vi "Filter Repeat Barrels.vi"(8 "error in (no error)":errorcluster, 10 "Barrel Array":T1(array[cluster])) -> (0 "error out":errorcluster, 2 "Observed LM Array":T1(array[cluster]))   [LabVIEW 2009]
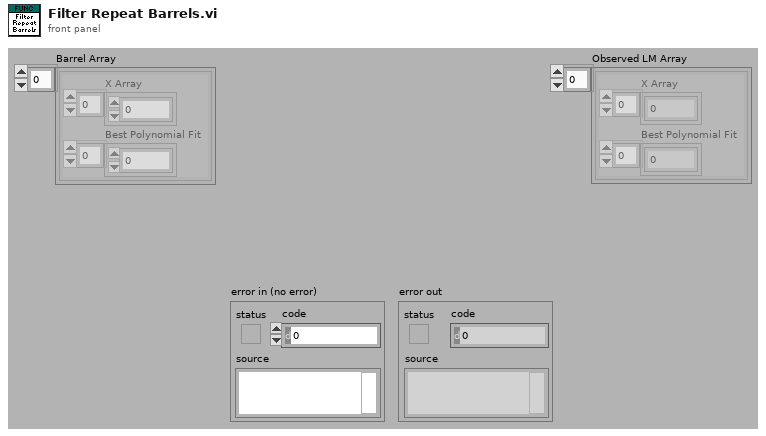
[diagram p1: front panel]
types:
  T1 = cluster{"X Array":dbl[], "Best Polynomial Fit":dbl[]}[]
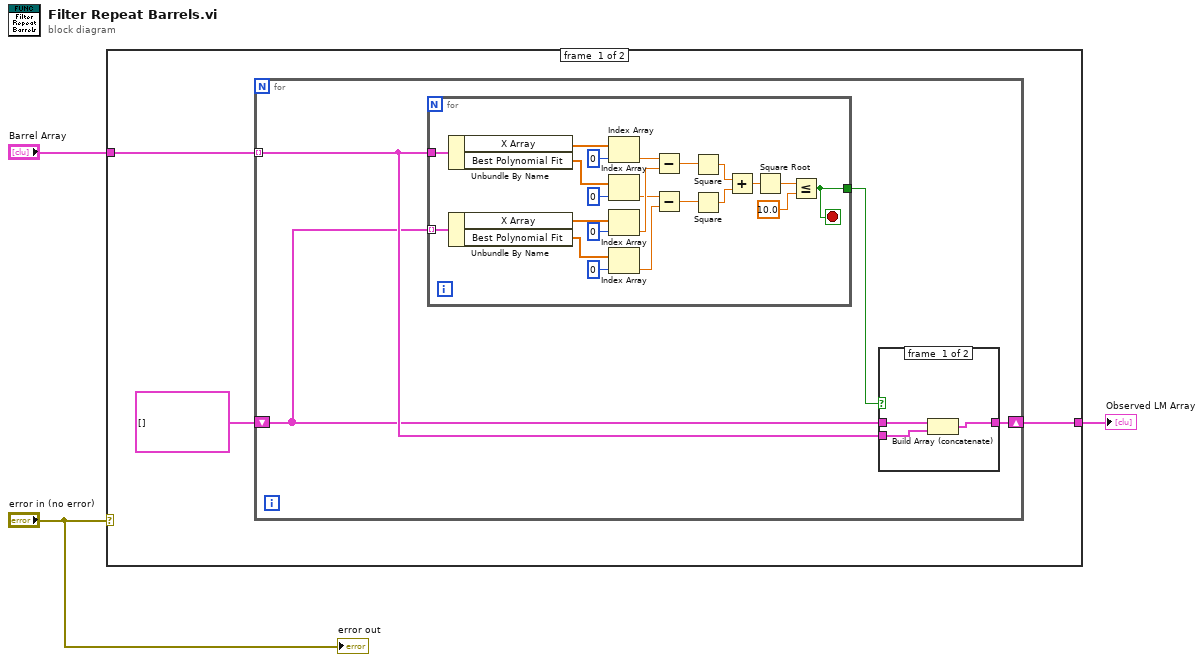
[diagram p0: block diagram]
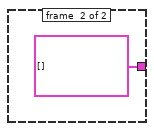
[diagram p3: hidden frame]
diagram:
  n1 = case shown="No Error" "error in (no error)" {
    tunnel: "Barrel Array" -> [w5 _]
    tunnel: [w4 T1 []] -> w2
    frame #0 {
      n2 = for {
        tunnel: w5 -> [w10] mode=indexing
        shift-right: [w7] -> w4
        shift-left: T1 [] -> [w8]
        n3 = for {
          tunnel: w8 -> [w35] mode=indexing
          tunnel: w10 -> [w36]
          tunnel: [w15] -> w9
          stop <- w15 stop-if-true
          n4 = Unbundle By Name(w36) -> ("X Array"=w27:dbl[], "Best Polynomial Fit"=w32:dbl[])
          n5 = Unbundle By Name(w35) -> ("X Array"=w29:dbl[], "Best Polynomial Fit"=w28:dbl[])
          n6 = Index Array(array=w27, index=0) -> (element=w26:dbl)
          n7 = Index Array(array=w32, index=0) -> (element=w24:dbl)
          n8 = Index Array(array=w29, index=0) -> (element=w25:dbl)
          n9 = Index Array(array=w28, index=0) -> (element=w23:dbl)
          n10 = Subtract(x=w26, y=w25) -> (x-y=w17:dbl)
          n11 = Subtract(x=w24, y=w23) -> (x-y=w16:dbl)
          n12 = Square(x=w17) -> (x^2=w18:dbl)
          n13 = Square(x=w16) -> (x^2=w19:dbl)
          n14 = Add(x=w18, y=w19) -> (x+y=w20:dbl)
          n15 = Square Root(x=w20) -> (sqrt(x)=w21:dbl)
          n16 = Less Or Equal?(x=w21, y=10.0) -> (x <= y?=w15:bool)
        }
        n17 = case shown="False" w9 {
          tunnel: w10 -> [w12 _]
          tunnel: w8 -> [w13 w14]
          tunnel: [w11 w14] -> w7
          frame #0 {
            n18 = Build Array (concatenate)(w13, w12) -> (w11:T1)
          }
          frame #1 {
          }
        }
      }
    }
    frame #1 {
    }
  }
  "Observed LM Array" <- w2
  "error out" <- "error in (no error)"
